vi "Create.vi"(5 "HttpRequestMessage in":refnum<class "HttpRequestMessage.lvclass">, 6 "Uri":refnum<k24>, 7 "Method [GET]":T1, 8 "error in (no error)":errorcluster, 11 "Address":string) -> (0 "error out":errorcluster, 3 "HttpRequestMessage out":refnum<class "HttpRequestMessage.lvclass">)   [LabVIEW 2018, in "LabVIEWHTTPClient_NET.lvlib" / "HttpRequestMessage.lvclass"]
uses:
  HttpRequestMessage.lvclass
  Types/method_enum.ctl
  System.Net.Http
  LabVIEWHTTPClient_NET/LabVIEWHTTPClient_NET.lvclass
  LabVIEWHTTPClient_NET/LabVIEWHTTPClient_NET.lvlib
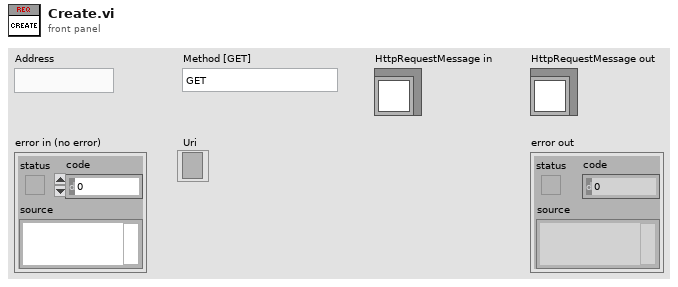
[diagram p1: front panel]
types:
  T1 = typedef "LabVIEWHTTPClient_NET.lvlib/method_enum.ctl" = enum16{"GET", "PUT", "POST", "DELETE", "HEAD", "TRACE", "SEND"}
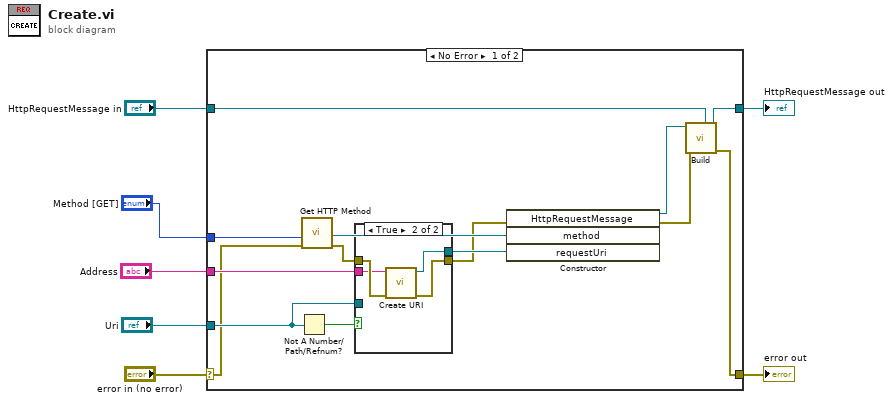
[diagram p0: block diagram]
diagram:
  n1 = case shown="No Error" "error in (no error)" {
    selector: "error in (no error)" -> [w12 w29]
    tunnel: [w10 w29] -> w6
    tunnel: [w13 w28] -> w4
    tunnel: "HttpRequestMessage in" -> [w8 w28]
    tunnel: "Method [GET]" -> [w17 _]
    tunnel: "Address" -> [w16 _]
    tunnel: "Uri" -> [w14 _]
    frame No Error {
      n2 = Not A Number/Path/Refnum?(number/path/refnum=w14) -> (NaN/Path/Refnum?=w15:bool)
      n3 = call "Get HTTP Method.vi"("Error In"=w12, "Enum"=w17) -> ("error out"=w20:errorcluster, "HTTPMethod"=w19:refnum<k24>)  [unwired: 8 in]
      n4 = case shown="True" w15 {
        tunnel: [w23 w24] -> w21
        tunnel: w20 -> [w22 w27]
        tunnel: [w22 w25] -> w18
        tunnel: w16 -> [_ w26]
        tunnel: w14 -> [w23 _]
        frame False {
        }
        frame True {
          n5 = call "Create URI.vi"("error in (no error)"=w27, "uriString"=w26) -> ("error out"=w25:errorcluster, ".NET Refnum out"=w24:refnum<k24>)  [unwired: 8 in]
        }
      }
      n6 = constructor class="HttpRequestMessage"(error in=w18, "method"=w19, "requestUri"=w21) -> (reference out=w9:refnum<k24>, error out=w11:errorcluster)  [unwired: 2 in, 3 out]
      n7 = call "Build.vi"("HttpRequestMessage in"=w8, "error in (no error)"=w11, "HttpRequestMessage"=w9) -> ("error out"=w10:errorcluster, "HttpRequestMessage out"=w13:refnum<class "HttpRequestMessage.lvclass">)  [unwired: 7 in]
    }
    frame Error {
    }
  }
  "error out" <- w6
  "HttpRequestMessage out" <- w4
